vi "Ref_Group_cntrl.vi"(0 "Group ch 4":refnum<vi>, 1 "Group ch 5":refnum<vi>, 2 "Group ch 6":refnum<vi>, 3 "Init":bool, 4 "Group ch 7":refnum<vi>, 5 "Group ch 8":refnum<vi>, 6 "Group ch 9":refnum<vi>, 7 "error in":errorcluster, 8 "Group ch 3":refnum<vi>, 9 "Group ch 10":refnum<vi>, 10 "Group ch 2":refnum<vi>, 11 "Group ch 11":refnum<vi>, 12 "Group ch 1":refnum<vi>, 13 "Group ch 12":refnum<vi>) -> (15 "Group ch 1 out":refnum<vi>, 16 "Group ch 12 out":refnum<vi>, 17 "Group ch 2 out":refnum<vi>, 18 "Group ch 11 out":refnum<vi>, 19 "Group ch 3 out":refnum<vi>, 20 "Group ch 10 out":refnum<vi>, 21 "Group ch 9 out":refnum<vi>, 22 "Group ch 8 out":refnum<vi>, 23 "Group ch 7 out":refnum<vi>, 24 "Group ch 6 out":refnum<vi>, 25 "Group ch 5 out":refnum<vi>, 26 "Group ch 4 out":refnum<vi>, 27 "error out":errorcluster)   [LabVIEW 2017]
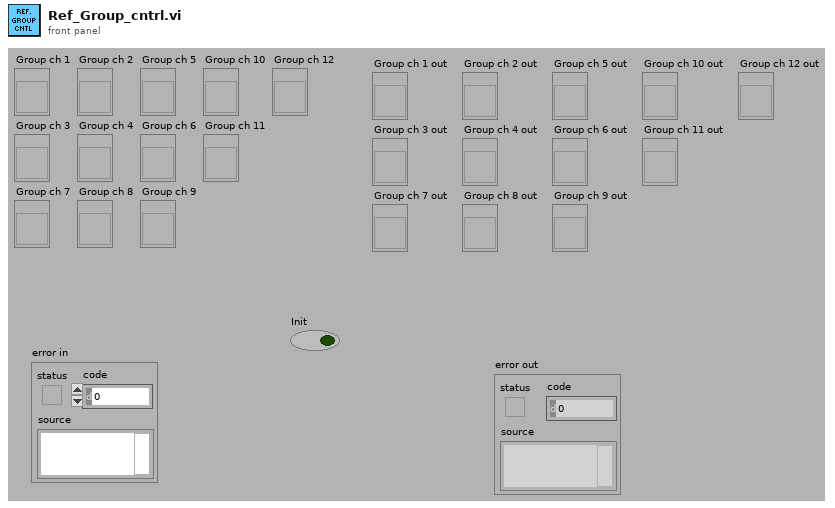
[diagram p1: front panel]
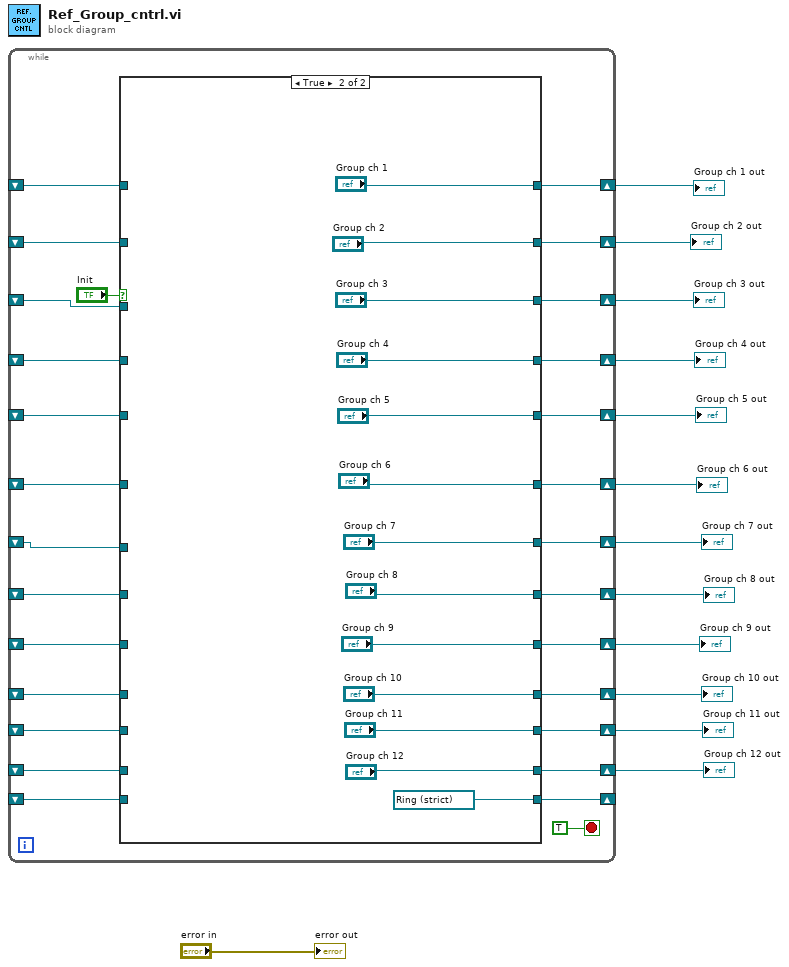
[diagram p0: block diagram]
diagram:
  n1 = while {
    shift-right: [w30] -> w13
    shift-left: _ -> [w36]
    shift-right: [w40] -> w12
    shift-left: _ -> [w35]
    shift-right: [w39] -> w11
    shift-left: _ -> [w34]
    shift-right: [w38] -> w10
    shift-left: _ -> [w33]
    shift-right: [w37] -> w9
    shift-left: _ -> [w32]
    shift-right: [w29] -> w8
    shift-left: _ -> [w28]
    shift-right: [w27] -> w7
    shift-left: _ -> [w26]
    shift-right: [w25] -> w6
    shift-left: _ -> [w19]
    shift-right: [w24] -> w5
    shift-left: _ -> [w18]
    shift-right: [w23] -> w4
    shift-left: _ -> [w17]
    shift-right: [w22] -> w3
    shift-left: _ -> [w16]
    shift-right: [w21] -> w2
    shift-left: _ -> [w15]
    shift-right: [w20] -> _
    shift-left: _ -> [w14]
    stop <- TRUE stop-if-true
    n2 = case shown="True" "Init" {
      tunnel: [w50 "Group ch 1"] -> w30
      tunnel: [w54 "Group ch 2"] -> w40
      tunnel: [w53 "Group ch 3"] -> w39
      tunnel: [w52 "Group ch 4"] -> w38
      tunnel: [w51 "Group ch 5"] -> w37
      tunnel: w36 -> [w50 _]
      tunnel: w35 -> [w54 _]
      tunnel: w34 -> [w53 _]
      tunnel: w33 -> [w52 _]
      tunnel: w32 -> [w51 _]
      tunnel: [w49 "Group ch 6"] -> w29
      tunnel: w28 -> [w49 _]
      tunnel: [w48 "Group ch 7"] -> w27
      tunnel: w26 -> [w48 _]
      tunnel: [w47 "Group ch 8"] -> w25
      tunnel: [w46 "Group ch 9"] -> w24
      tunnel: [w45 "Group ch 10"] -> w23
      tunnel: [w44 "Group ch 11"] -> w22
      tunnel: [w43 "Group ch 12"] -> w21
      tunnel: [w42 refnum<vi> refnum ("Group ch 13")] -> w20
      tunnel: w19 -> [w47 _]
      tunnel: w18 -> [w46 _]
      tunnel: w17 -> [w45 _]
      tunnel: w16 -> [w44 _]
      tunnel: w15 -> [w43 _]
      tunnel: w14 -> [w42 _]
      frame False {
      }
      frame True {
      }
    }
  }
  "Group ch 1 out" <- w13
  "Group ch 2 out" <- w12
  "Group ch 3 out" <- w11
  "Group ch 4 out" <- w10
  "Group ch 5 out" <- w9
  "Group ch 6 out" <- w8
  "Group ch 7 out" <- w7
  "Group ch 8 out" <- w6
  "Group ch 9 out" <- w5
  "Group ch 10 out" <- w4
  "Group ch 11 out" <- w3
  "Group ch 12 out" <- w2
  "error out" <- "error in"
